vi "iMic-GUI.vi"() -> ()   [LabVIEW 2011]
uses:
  <vilib>/event_ctls.llb/lveventtype.ctl
  <vilib>/Utility/inputDevices.llb/closeMouse.vi
  <vilib>/Utility/inputDevices.llb/mouseAcquire.vi
panel:
  out "obj.mag":i32=20
  in  "Stage control":enum32{"xy", "Steps", "Setup", "Status"}(tab)
  in  "Cluster":T1
  in  "Stepsize [mm]":dbl(slide)=0.4602583962404807 scale=0.01..5.0
  in  "scale":T2(array[cluster])=[{"last value"=0.0, "min."=0.0, "max"=7.0, "min.step"=0.0005, "String"="stage.z"}, {"last value"=0.18000000000000002, "min."=0.0, "max"=0.25, "min.step"=1e-05, "String"="stage.piezo"}]
  in  "Objektiv Offsets":cluster{"x":dbl, "y":dbl, "z":dbl}[](array[cluster]) {"z" format="%#.3p"; "y" format="%#.3p"; "x" format="%#.3p"}
  in  "xy Angle":dbl
  in  "clockwise":bool
  out "stop 2":bool
  out "scroll timed out":bool=TRUE
  out "Mouse inside?":T3
  out "scroll units^3":dbl
  in  "Pos [mm]":cluster{"x":dbl, "y":dbl}={"x"=56.550000000000004, "y"=34.7} {"x" format="%.4f"; "y" format="%.4f"}
  in  "Slider 2":sgl(ring) caption="filter.f2" items=["Kamera", "offen", "offen"]
  in  "Slider 1":sgl(ring) caption="filter.f1" items=["2Photon", "offen", "LED"]
  in  "Objective":u16(ring) items=["4x/0.1", "60x/1.2W", "60x0.9W_LD", "44x/1.3"]
  in  "z[mm]":dbl(slide) min=0.0 max=21.5 step=1e-05 scale=0.0..21.5 scale format="%#.3f"
  in  "Motor":bool
  in  "stop":bool
  # "0:Stepper\n1: Piezo"
  # "add this\nto variables!"
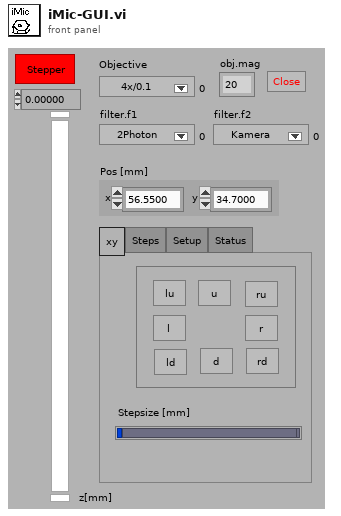
[diagram p1: front panel]
types:
  T1 = cluster{"r":bool, "ru":bool, "u":bool, "lu":bool, "l":bool, "ld":bool, "d":bool, "rd":bool}
  T2 = cluster{"last value":dbl, "min.":dbl, "max":dbl, "min.step":dbl, "String":string}[]
  T3 = typedef "lveventtype.ctl" = enum32{"Null", "Timeout", "App Instance Close", "App Instance Close?", "Autoscale Range Change", "Cell Edit", "Cell Edit?", "Cursor Grab", "Cursor Grab?", "Cursor Move", "Cursor Release", "Data Change", "Direction Change", "Display State Change", "Drag Ended", "Drag Enter", "Drag Leave", "Drag Over", "Drag Source Update", "Drag Starting", "Drag Starting?", "Drop", "Exec State Change", "Key Down", "Key Down?", "Key Repeat", "Key Repeat?", "Key Up", "Listbox Double Click", "Menu Activation?", "Menu Selection (App)", "Menu Selection? (App)", "Menu Selection (User)", "Mouse Down", "Mouse Down?", "Mouse Enter", "Mouse Leave", "Mouse Move", "Mouse Up", "NI Security User Change (App)", "Pane Size", "Panel Close", "Panel Close?", "Panel Resize", "Plot Attribute Change", "Scale Range Change", "Shortcut Menu Activation?", "Shortcut Menu Selection (App)", "Shortcut Menu Selection? (App)", "Shortcut Menu Selection (User)", "Tree Double Click", "Tree Drag", "Tree Drag?", "Tree Drop", "Tree Drop?", "Tree Item Close", "Tree Item Close?", "Tree Item Open", "Tree Item Open?", "Value Change"}
  T4 = enum16{"None/#Datasets", "Clear", "TagValueOf#", "AddValues", "ReadValue", "ChangeValue", "Get all"}
  T5 = cluster{"default value 1":dbl, "default value 1":dbl, "default value 1":dbl}
  T6 = cluster{"last value":dbl, "min.":dbl, "max":dbl, "min.step":dbl, "String":string}
  T7 = cluster{"Horizontal":i32, "Vertical":i32, "Scrolling":i32}
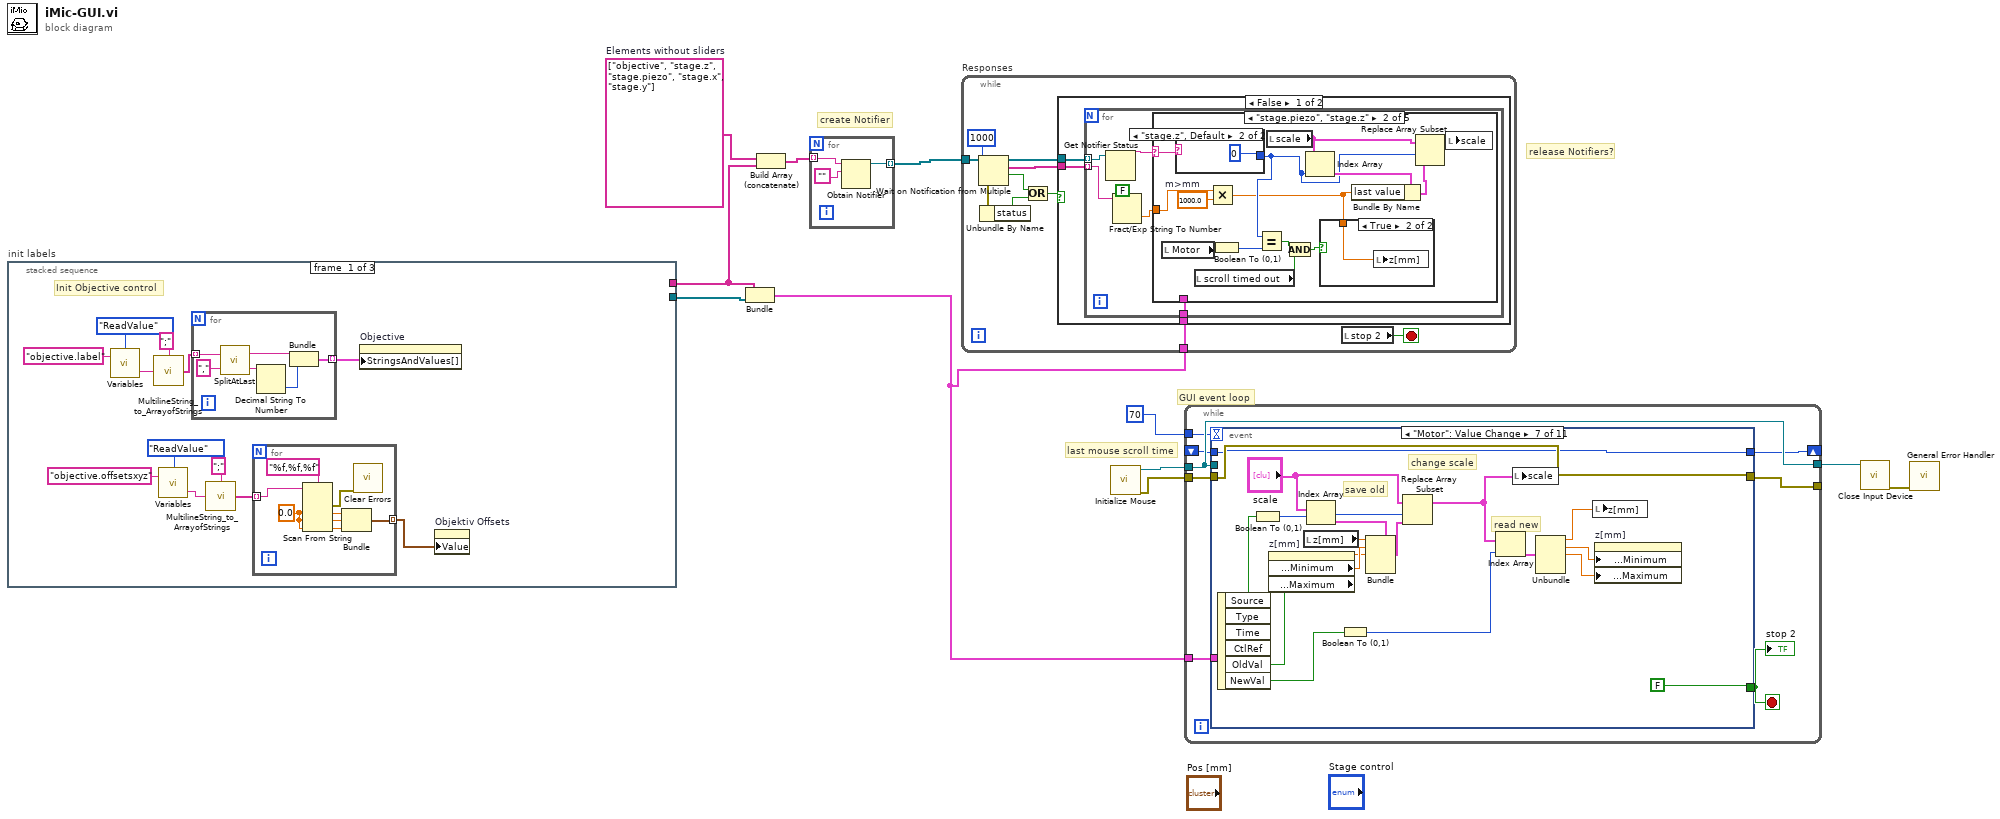
[diagram p0: block diagram]
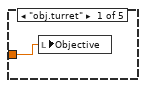
[diagram p2: hidden frame]
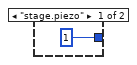
[diagram p4: hidden frame]
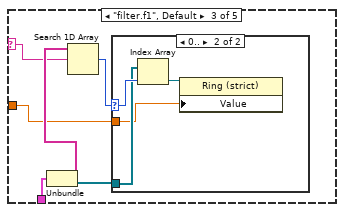
[diagram p5: hidden frame]
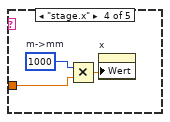
[diagram p7: hidden frame]
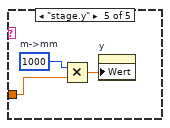
[diagram p8: hidden frame]
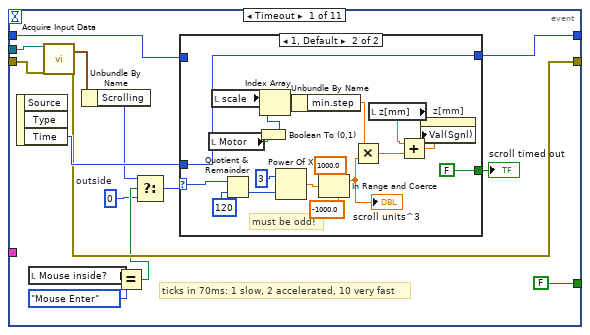
[diagram p10: hidden frame]
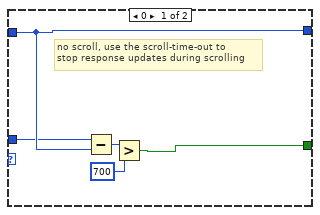
[diagram p11: hidden frame]
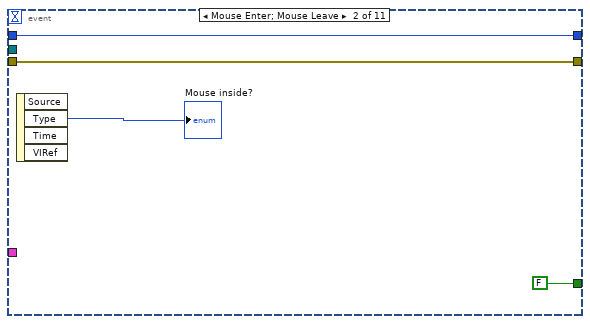
[diagram p12: hidden frame]
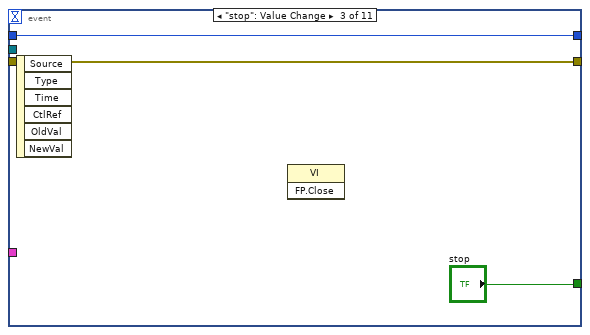
[diagram p13: hidden frame]
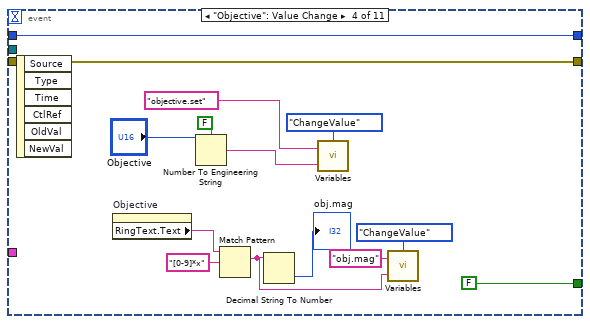
[diagram p14: hidden frame]
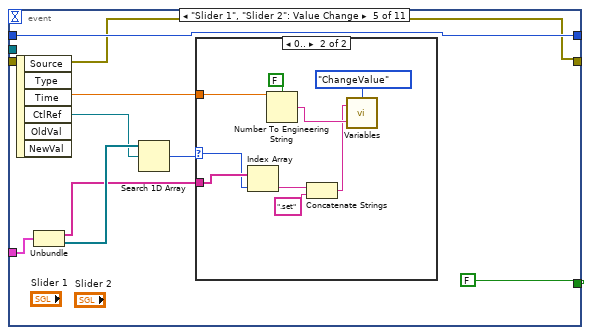
[diagram p15: hidden frame]
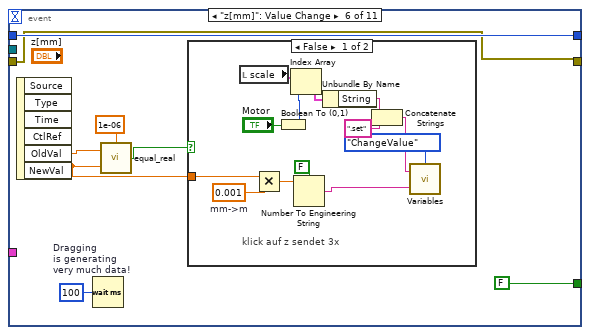
[diagram p17: hidden frame]
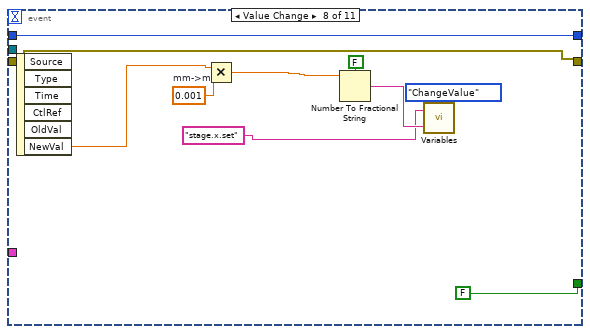
[diagram p19: hidden frame]
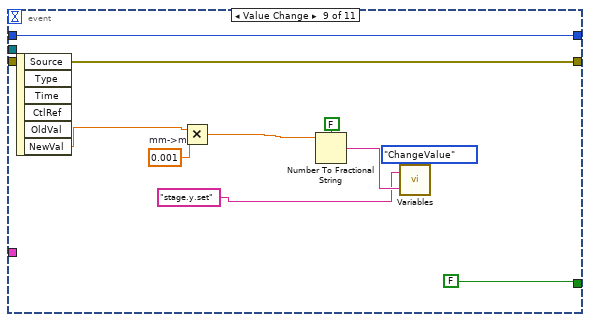
[diagram p20: hidden frame]
diagram:
  w11 = string[] ["objective", "stage.z", "stage.piezo", "stage.x", "stage.y"]  # Elements without sliders
  # "last mouse scroll time"
  # "release Notifiers?"
  # "create Notifier"
  # "GUI event loop"
  n1 = stacked-sequence "init labels" {
    tunnel: [_ w42 _] -> w9
    tunnel: [_ w41 _] -> w7
    frame #0 {
      # "Init Objective control"
      n2 = call "Variables.vi"("Tag in"="objective.label", "Command"=T4."ReadValue") -> ("value out"=w20:string)  [unwired: 1 in, 2 out]
      n3 = call "MultilineString_to_ArrayofStrings.vi"("String 1"=w20, "NewLineString"=";") -> ("String Array"=w21:string[])
      n4 = call "Variables.vi"("Tag in"="objective.offsetsxyz", "Command"=T4."ReadValue") -> ("value out"=w14:string)  [unwired: 1 in, 2 out]
      n5 = for {
        tunnel: w21 -> [w37] mode=indexing
        tunnel: [w32] -> w23 mode=indexing
        n6 = call "SplitAtLast.vi"("search char"=",", "In-String"=w37) -> ("end"=w35:string, "Front (default)"=w34:string)
        n7 = Decimal String To Number(string=w35) -> (number=w33:i32)  [unwired: 3 out]
        n8 = Bundle("Front (default)"=w34, w33) -> (w32:cluster{"Front (default)":string, i32})  [unwired: 1 out]
      }
      n9 = call "MultilineString_to_ArrayofStrings.vi"("String 1"=w14, "NewLineString"=";") -> ("String Array"=w13:string[])
      n10 = for {
        tunnel: w13 -> [w25] mode=indexing
        tunnel: [w24] -> w12 mode=indexing
        w27 = 0.0 ("default value 1")
        n11 = Scan From String(format string="%f,%f,%f" ("Format-String"), input string=w25, default 1=w27, default 2=w27, default 3=w27) -> (error out=w26:errorcluster, output 1=w30:dbl, output 2=w29:dbl, output 3=w28:dbl)  [unwired: 2 in, 2 out]
        n12 = Bundle("default value 1"=w30, "default value 1"=w29, "default value 1"=w28) -> (w24:T5)  [unwired: 1 out]
        n13 = call <vilib>:"Clear Errors.vi"("error in (no error)"=w26) -> ()  [unwired: 7 out]
      }
      n14 = property on="Objective" class="Ring (strict)"("StringsAndValues[]"=w23) -> ()  [unwired: 2 in, 2 out]
      n15 = property on="Objektiv Offsets" class="Arr (strict)"("Value"=w12) -> ()  [unwired: 2 in, 2 out]
    }
    frame #1 {
      # "Init filter slider control"
      n16 = call "Variables.vi"("Tag in"="filter.tags", "Command"=T4."ReadValue") -> ("value out"=w44:string)  [unwired: 1 in, 2 out]
      n17 = call "MultilineString_to_ArrayofStrings.vi"("String 1"=w44, "NewLineString"=",") -> ("String Array"=w42:string[])
      n18 = control-ref of="Slider 2"() -> (w40:refnum<vi>)
      n19 = control-ref of="Slider 1"() -> (w39:refnum<vi>)
      n20 = Build Array(w39, w40) -> (w38:refnum<vi>[])
      n21 = for {
        tunnel: w42 -> [w50] mode=indexing
        tunnel: w38 -> [w48] mode=indexing
        tunnel: [w47] -> w41 mode=indexing
        n22 = Concatenate Strings(w50, ".label" ("string")) -> (w51:string)
        n23 = call "Variables.vi"("Tag in"=w51, "Command"=T4."ReadValue") -> ("value out"=w55:string)  [unwired: 1 in, 2 out]
        n24 = call "MultilineString_to_ArrayofStrings.vi"("String 1"=w55, "NewLineString"=";") -> ("String Array"=w54:string[])
        n25 = for {
          tunnel: w54 -> [w64] mode=indexing
          tunnel: [w59] -> w53 mode=indexing
          n26 = call "SplitAtLast.vi"("search char"=",", "In-String"=w64) -> ("end"=w62:string, "Front (default)"=w61:string)
          n27 = Fract/Exp String To Number(use system decimal point (T)=FALSE, string=w62) -> (number=w60:dbl)  [unwired: 3 out]
          n28 = Bundle("Front (default)"=w61, w60) -> (w59:cluster{"Front (default)":string, dbl})  [unwired: 1 out]
        }
        n29 = property on="Property Node" class="Ring (strict)"(reference=w48, "StringsAndValues[]"=w53, "Visible"=TRUE, "Caption.Text"=w50) -> (reference out=w47:refnum<vi>)  [unwired: 1 in, 1 out]
      }
    }
    frame #2 {
      # "it would be good to Read/update all elements"
      # "update obj.mag\nan external change in Objective.set will probably forget to set obj.mag?"
      n30 = call "Variables.vi"("Tag in"="stage.z", "Command"=T4."ReadValue") -> ("value out"=w70:string)  [unwired: 1 in, 2 out]
      n31 = call "Variables.vi"("Tag in"="obj.mag", "Command"=T4."ReadValue") -> ("value out"=w75:string)  [unwired: 1 in, 2 out]
      n32 = Fract/Exp String To Number(use system decimal point (T)=TRUE, string=w70) -> (number=w69:dbl)  [unwired: 3 out]
      n33 = Decimal String To Number(string=w75, default (0L)=60 ("default (0 I32)")) -> (number=w74:i32)  [unwired: 2 out]
      n34 = local write "obj.mag"(w74) -> ()
      n35 = Multiply(x=1000.0, y=w69) -> (x*y=w67:dbl)
      n36 = local write "z[mm]"(w67) -> ()
      n37 = local write "stop 2"(FALSE ("stop 2")) -> ()
    }
  }
  n38 = Bundle("String Array"=w9, w7) -> (w8:cluster{"String Array":string[], refnum<vi>[]})  [unwired: 1 out]
  n39 = Build Array (concatenate)(w11, w9) -> (w10:string[])
  n40 = for {
    tunnel: w10 -> [w79] mode=indexing
    tunnel: [w80] -> w6 mode=indexing
    n41 = Obtain Notifier(name (unnamed)=w79, notification data type="") -> (notifier out=w80:refnum<notifier>)  [unwired: 2 in, 2 out]
  }
  n42 = while "Responses" {
    tunnel: w6 -> [w90]
    tunnel: w8 -> [w82]
    stop <- w81 stop-if-true
    n43 = Wait on Notification from Multiple(0:w90, 2:1000 ("timeout in ms (-1)")) -> (8:w85:refnum<notifier>[], 9:w84:string[], 10:w86:bool, 11:w88:errorcluster)  [unwired: 1 in, 1 out]
    n44 = Unbundle By Name(w88) -> ("status"=w87:bool)
    n45 = Or(x=w86, y=w87) -> (x .or. y?=w83:bool)
    n46 = case shown="False" w83 {
      tunnel: w85 -> [w93 _]
      tunnel: w84 -> [w92 _]
      tunnel: w82 -> [w91 _]
      frame False {
        n47 = for {
          tunnel: w93 -> [w99] mode=indexing
          tunnel: w92 -> [w97] mode=indexing
          tunnel: w91 -> [w94]
          n48 = Get Notifier Status(notifier=w99) -> (notifier name=w98:string)  [unwired: 1 in, 4 out]
          n49 = Fract/Exp String To Number(use system decimal point (T)=FALSE, string=w97) -> (number=w95:dbl)  [unwired: 3 out]
          n50 = case shown="\"stage.piezo\", \"stage.z\"" w98 {
            selector: w98 -> [_ w114 w120 _ _]
            tunnel: w95 -> [w100 w106 w118 w129 w133]
            tunnel: w94 -> [_ _ w123 _ _]
            frame "obj.turret" {
              n51 = local write "Objective"(w100) -> ()
            }
            frame "stage.piezo", "stage.z" {
              w104 = 1000.0  # m>mm
              n52 = local read "Motor"() -> (w103:bool)
              n53 = case shown="\"stage.z\", Default" w114 {
                tunnel: [1 0] -> w108
                frame "stage.piezo" {
                }
                frame "stage.z", Default {
                }
              }
              n54 = local read "scroll timed out"() -> (w101:bool)
              n55 = Multiply(x=w106, y=w104) -> (x*y=w105:dbl)
              n56 = Boolean To (0,1)(Boolean=w103) -> (0, 1=w109:i16)
              n57 = Equal?(x=w108, y=w109) -> (x = y?=w107:bool)
              n58 = local read "scale"() -> (w112:T2)
              n59 = And(x=w107, y=w101) -> (x .and. y?=w102:bool)
              n60 = Index Array(array=w112, index=w108) -> (element=w113:T6)
              n61 = case shown="True" w102 {
                tunnel: w105 -> [_ w115]
                frame False {
                }
                frame True {
                  n62 = local write "z[mm]"(w115) -> ()
                }
              }
              n63 = Bundle By Name(cluster=w113, "last value"=w105) -> (w111:T6)
              n64 = Replace Array Subset(array=w112, new element=w111, index=w108) -> (w110:T2)
              n65 = local write "scale"(w110) -> ()
            }
            frame "filter.f1", Default {
              n66 = Unbundle(w123) -> ("String Array"=w121:string[], w122:refnum<vi>[])
              n67 = Search 1D Array(1D array=w121, element=w120) -> (index of element=w119:i32)  [unwired: 1 out]
              n68 = case shown="0.." w119 {
                selector: w119 -> [_ w127]
                tunnel: w122 -> [_ w126]
                tunnel: w118 -> [_ w124]
                frame -1, Default {
                }
                frame 0.. {
                  n69 = Index Array(array=w126, index=w127) -> (element=w125:refnum<vi>)
                  n70 = property on="Property Node" class="Ring (strict)"(reference=w125, "Value"=w124) -> ()  [unwired: 1 in, 2 out]
                }
              }
            }
            frame "stage.x" {
              w130 = 1000  # m->mm
              n71 = Multiply(x=w130, y=w129) -> (x*y=w128:dbl)
              n72 = property on="x" class="DigNum (strict)"("Wert"=w128) -> ()  [unwired: 2 in, 2 out]
            }
            frame "stage.y" {
              w132 = 1000  # m->mm
              n73 = Multiply(x=w132, y=w133) -> (x*y=w131:dbl)
              n74 = property on="y" class="DigNum (strict)"("Wert"=w131) -> ()  [unwired: 2 in, 2 out]
            }
          }
        }
      }
      frame True {
        # "err or timeout"
      }
    }
    n75 = local read "stop 2"() -> (w81:bool)
  }
  n76 = call <vilib>:"Initialize Mouse.vi"() -> ("error out"=w2:errorcluster, "device ID"=w4:refnum<k1>)  [unwired: 1 in, 9 out]
  n77 = while {
    tunnel: w8 -> [w141]
    tunnel: w4 -> [w140]
    tunnel: [w140] -> w3
    tunnel: w2 -> [w139]
    tunnel: [w138] -> _
    shift-right: [w136] -> _
    shift-left: _ -> [w137]
    tunnel: u32 70 ("milliseconds to wait") -> [w134]
    stop <- w135 stop-if-true
    n78 = event shown="[6] \"Motor\": Value Change" {
      selector: _ -> [_ _ _ _ _ _ _ _ _ _ _]
      dyn-events: _ -> [_ _ _ _ _ _ _ _ _ _ _]
      timeout: w134 -> [_ _ _ _ _ _ _ _ _ _ _]
      tunnel: [FALSE ("stop") FALSE ("stop") "stop" FALSE FALSE FALSE FALSE ("stop") FALSE FALSE ("stop") FALSE ("stop") FALSE ("stop")] -> w135
      tunnel: w141 -> [_ _ _ _ w207 _ _ _ _ _ _]
      tunnel: w140 -> [w156 _ _ _ _ _ _ _ _ _ _]
      tunnel: w139 -> [w155 w180 w184 w187 w201 w219 w241 w259 w268 w278 w317]
      tunnel: [w148 w180 w184 w187 w201 w219 w241 w259 w268 w278 w317] -> w138
      tunnel: w137 -> [w152 w181 w185 w188 w202 w220 w240 w258 w269 w279 w316]
      tunnel: [w153 w181 w185 w188 w202 w220 w240 w258 w269 w279 w316] -> w136
      event Timeout {
        w142 = 0  # outside
        # "ticks in 70ms: 1 slow, 2 accelerated, 10 very fast"
        n79 = event-data() -> ("Time"=w151:u32)  [unwired: 3 out]
        n80 = local read "Mouse inside?"() -> (w147:T3)
        n81 = call-poly <vilib>:"Acquire Input Data.vi"("device ID"=w156, "error in (no error)"=w155) -> ("axis info"=w154:T7, "error out"=w148:errorcluster)  [unwired: 1 in, 15 out]
        n82 = Unbundle By Name(w154) -> ("Scrolling"=w144:i32)
        n83 = Equal?(x=w147, y=lveventtype."Mouse Enter" ("Type")) -> (x = y?=w145:bool)
        n84 = Select(t=w144, s=w145, f=w142) -> (s? t:f=w143:i32)
        n85 = case shown="1, Default" w143 {
          selector: w143 -> [_ w171]
          tunnel: w152 -> [w161 _]
          tunnel: [w161 w172] -> w153
          tunnel: w151 -> [w158 w172]
          tunnel: [w157 FALSE] -> w149
          frame 0 {
            # "no scroll, use the scroll-time-out to\nstop response updates during scrolling"
            n86 = Subtract(x=w158, y=w161) -> (x-y=w160:u32)
            n87 = Greater?(x=w160, y=u32 700) -> (0:w157:bool)
          }
          frame 1, Default {
            # "must be odd!"
            n88 = local read "Motor"() -> (w176:bool)
            n89 = local read "scale"() -> (w177:T2)
            n90 = Quotient & Remainder(x=w171, y=120) -> (floor(x/y)=w169:i32)  [unwired: 1 out]
            n91 = Boolean To (0,1)(Boolean=w176) -> (0, 1=w174:i16)
            n92 = Index Array(array=w177, index=w174) -> (element=w175:T6)
            n93 = Power Of X(1:w169, 2:3 ("y")) -> (0:w167:dbl)
            n94 = Unbundle By Name(w175) -> ("min.step"=w163:dbl)
            n95 = In Range and Coerce(upper limit=1000.0, x=w167, lower limit=-1000.0) -> (coerced(x)=w166:dbl)  [unwired: 1 out]
            "scroll units^3" <- w166
            n96 = Multiply(x=w163, y=w166) -> (x*y=w179:dbl)
            n97 = local read "z[mm]"() -> (w178:dbl)
            n98 = Add(x=w178, y=w179) -> (x+y=w173:dbl)
            n99 = property on="z[mm]" class="Slide (strict)"("Val(Sgnl)"=w173) -> ()  [unwired: 2 in, 2 out]
          }
        }
        "scroll timed out" <- w149
      }
      event Mouse Enter; Mouse Leave {
        n100 = event-data() -> ("Type"=→"Mouse inside?":T3)  [unwired: 4 out]
      }
      event "stop": Value Change {
        n101 = event-data() -> ()  [unwired: 7 out]
        n102 = invoke class="VI" method="FP.Close"() -> ()  [unwired: 3 in, 3 out]
      }
      event "Objective": Value Change {
        n103 = event-data() -> ()  [unwired: 7 out]
        n104 = property on="Objective" class="Ring (strict)"() -> ("RingText.Text"=w193:string)  [unwired: 2 in, 2 out]
        n105 = Number To Engineering String(1:FALSE ("use system decimal point (T)"), 4:"Objective") -> (0:w197:string)  [unwired: 2 out]
        n106 = Match Pattern(string=w193, regular expression="[0-9]*x" ("regulärer Ausdruck")) -> (match substring=w190:string)  [unwired: 4 out]
        n107 = Decimal String To Number(string=w190) -> (number=→"obj.mag":i32)  [unwired: 3 out]
        n108 = call "Variables.vi"("value"=w197, "Tag in"="objective.set", "Command"=T4."ChangeValue") -> ()  [unwired: 3 out]
        n109 = call "Variables.vi"("value"=w190, "Tag in"="obj.mag", "Command"=T4."ChangeValue") -> ()  [unwired: 3 out]
      }
      event "Slider 1", "Slider 2": Value Change {
        n110 = event-data() -> ("CtlRef"=w205:refnum<vi>, "NewVal"=w209:sgl)  [unwired: 5 out]
        n111 = Unbundle(w207) -> ("String Array"=w203:string[], w206:refnum<vi>[])
        n112 = Search 1D Array(1D array=w206, element=w205) -> (index of element=w204:i32)  [unwired: 1 out]
        n113 = case shown="0.." w204 {
          selector: w204 -> [_ w213]
          tunnel: w209 -> [_ w218]
          tunnel: w203 -> [_ w214]
          frame -1, Default {
          }
          frame 0.. {
            n114 = Index Array(array=w214, index=w213) -> (element=w212:string)
            n115 = Number To Engineering String(1:FALSE ("use system decimal point (T)"), 4:w218) -> (0:w217:string)  [unwired: 2 out]
            n116 = Concatenate Strings(w212, ".set" ("string")) -> (w211:string)
            n117 = call "Variables.vi"("value"=w217, "Tag in"=w211, "Command"=T4."ChangeValue") -> ()  [unwired: 3 out]
          }
        }
      }
      event "z[mm]": Value Change {
        w225 = u32 100  # Dragging is generating very much data!
        n118 = event-data() -> ("OldVal"=w224:dbl, "NewVal"=w223:dbl)  [unwired: 5 out]
        n119 = Wait (ms)(milliseconds to wait=w225) -> ()  [unwired: 1 out]
        n120 = call "equal_real.vi"("max rel deviation"=1e-06, "b"=w223, "a"=w224) -> ("Equal"=w222:bool)
        n121 = case shown="False" w222 {
          tunnel: w223 -> [w227 _]
          frame False {
            w234 = 0.001  # mm->m
            # "klick auf z sendet 3x"
            n122 = local read "scale"() -> (w237:T2)
            n123 = Multiply(x=w227, y=w234) -> (x*y=w233:dbl)
            n124 = Boolean To (0,1)(Boolean="Motor") -> (0, 1=w235:i16)
            n125 = Index Array(array=w237, index=w235) -> (element=w236:T6)
            n126 = Number To Engineering String(1:FALSE ("use system decimal point (T)"), 4:w233) -> (0:w229:string)  [unwired: 2 out]
            n127 = Unbundle By Name(w236) -> ("String"=w231:string)
            n128 = Concatenate Strings(w231, ".set" ("string")) -> (w232:string)
            n129 = call "Variables.vi"("value"=w229, "Tag in"=w232, "Command"=T4."ChangeValue") -> ()  [unwired: 3 out]
          }
          frame True {
          }
        }
      }
      event "Motor": Value Change {
        # "change scale"
        # "read new"
        # "save old"
        n130 = event-data() -> ("OldVal"=w253:bool, "NewVal"=w257:bool)  [unwired: 5 out]
        n131 = Boolean To (0,1)(Boolean=w253) -> (0, 1=w245:i16)
        n132 = property on="z[mm]" class="Slide (strict)"() -> ("Skalierung.Bereich:Minimum"=w250:dbl, "Skalierung.Bereich:Maximum"=w249:dbl)  [unwired: 2 in, 2 out]
        n133 = local read "z[mm]"() -> (w251:dbl)
        n134 = Index Array(array="scale", index=w245) -> (element=w252:T6)
        n135 = Boolean To (0,1)(Boolean=w257) -> (0, 1=w244:i16)
        n136 = Bundle(cluster=w252, "last value"=w251, "min."=w250, "max"=w249) -> (w255:T6)  [unwired: 2 out]
        n137 = Replace Array Subset(array="scale", new element=w255, index=w245) -> (w243:T2)
        n138 = Index Array(array=w243, index=w244) -> (element=w256:T6)
        n139 = local write "scale"(w243) -> ()
        n140 = Unbundle(w256) -> ("last value"=w242:dbl, "min."=w248:dbl, "max"=w247:dbl)  [unwired: 2 out]
        n141 = local write "z[mm]"(w242) -> ()
        n142 = property on="z[mm]" class="Slide (strict)"("Skalierung.Bereich:Minimum"=w248, "Skalierung.Bereich:Maximum"=w247) -> ()  [unwired: 2 in, 2 out]
      }
      event "Pos [mm].x": Value Change {
        w266 = 0.001  # mm->m
        n143 = event-data() -> ("NewVal"=w264:dbl)  [unwired: 6 out]
        n144 = Multiply(x=w264, y=w266) -> (x*y=w267:dbl)
        n145 = Number To Fractional String(use system decimal point (T)=FALSE, number=w267) -> (F-format string=w262:string)  [unwired: 2 out]
        n146 = call "Variables.vi"("value"=w262, "Tag in"="stage.x.set" ("Tag"), "Command"=T4."ChangeValue") -> ()  [unwired: 3 out]
      }
      event "Pos [mm].y": Value Change {
        w276 = 0.001  # mm->m
        n147 = event-data() -> ("NewVal"=w271:dbl)  [unwired: 6 out]
        n148 = Multiply(x=w271, y=w276) -> (x*y=w277:dbl)
        n149 = Number To Fractional String(use system decimal point (T)=FALSE, number=w277) -> (F-format string=w274:string)  [unwired: 2 out]
        n150 = call "Variables.vi"("value"=w274, "Tag in"="stage.y.set" ("Tag"), "Command"=T4."ChangeValue") -> ()  [unwired: 3 out]
      }
      event "Cluster": Value Change {
        w294 = 0.001  # mm->m
        # "anordung: index*45=winkel!"
        n151 = event-data() -> ("OldVal"=w310:T1)  [unwired: 6 out]
        n152 = Not Equal?(x=w310, y="Cluster") -> (x != y?=w309:T1)
        n153 = Cluster To Array(cluster=w309) -> (array=w308:bool[])
        n154 = Select(t=-1.0, s="clockwise", f=1.0) -> (s? t:f=w283:dbl)
        n155 = Search 1D Array(1D array=w308, element=TRUE ("Element")) -> (index of element=w306:i32)  [unwired: 1 out]
        n156 = Multiply(x=45, y=w306) -> (x*y=w305:i32)
        n157 = Multiply(x=w305, y=w283) -> (x*y=w284:dbl)
        n158 = Divide(x=3.141592653589793, y=180.0) -> (x/y=w285:dbl)
        n159 = Add(x=w284, y="xy Angle") -> (x+y=w282:dbl)
        n160 = Multiply(x=w282, y=w285) -> (x*y=w292:dbl)
        n161 = local read "Pos [mm]"() -> (w299:cluster{"x":dbl, "y":dbl})
        n162 = Cosine(x=w292) -> (cos(x)=w302:dbl)
        n163 = Sine(x=w292) -> (sin(x)=w301:dbl)
        n164 = Build Array(w302, w301) -> (w300:dbl[])
        n165 = Cluster To Array(cluster=w299) -> (array=w298:dbl[])
        n166 = Multiply(x=w300, y="Stepsize [mm]") -> (x*y=w303:dbl[])
        n167 = Add(x=w303, y=w298) -> (x+y=w296:dbl[])
        n168 = Multiply(x=w294, y=w296) -> (x*y=w295:dbl[])
        n169 = for {
          tunnel: w295 -> [w311] mode=indexing
          tunnel: string[] ["stage.x.set", "stage.y.set"] -> [w312] mode=indexing
          n170 = Number To Fractional String(use system decimal point (T)=FALSE, number=w311) -> (F-format string=w315:string)  [unwired: 2 out]
          n171 = call "Variables.vi"("value"=w315, "Tag in"=w312, "Command"=T4."ChangeValue") -> ()  [unwired: 3 out]
        }
      }
      event "Objektiv Offsets": Value Change {
        n172 = event-data() -> ("OldVal"=w319:cluster{"x":dbl, "y":dbl, "z":dbl}[], "NewVal"=w318:cluster{"x":dbl, "y":dbl, "z":dbl}[])  [unwired: 5 out]
        n173 = for {
          tunnel: w319 -> [w324] mode=indexing
          tunnel: w318 -> [w322] mode=indexing
          i -> [w321]
          n174 = Not Equal?(x=w324, y=w322) -> (x != y?=w323:bool)
          n175 = case shown="True" w323 {
            tunnel: w322 -> [_ w335]
            tunnel: w321 -> [_ w330]
            frame False {
            }
            frame True {
              n176 = Unbundle(w335) -> ("x"=w334:dbl, "y"=w333:dbl, "z"=w332:dbl)
              n177 = Number To Decimal String(number=w330) -> (decimal integer string=w329:string)  [unwired: 1 out]
              n178 = Format Into String(format string="%f,%f,%f" ("Format-String"), w334, w333, w332) -> (resulting string=w326:string)  [unwired: 2 in, 1 out]
              n179 = Concatenate Strings("obj.offsetxyz." ("Tag in"), w329) -> (w327:string)
              n180 = call "Variables.vi"("value"=w326, "Tag in"=w327, "Command"=T4."ChangeValue") -> ()  [unwired: 3 out]
            }
          }
        }
      }
    }
    "stop 2" <- w135
  }
  n181 = call-poly <vilib>:"Close Input Device.vi"("device ID"=w3) -> ("error out"=w5:errorcluster)  [unwired: 1 in, 8 out]
  n182 = call <vilib>:"General Error Handler.vi"("error in (no error)"=w5) -> ()  [unwired: 1 in, 14 out]
